vi "Circle_Geometry_Template.vi"(4 "Radius":dbl) -> (0 "Area":dbl, 1 "Circumference":dbl, 2 "Diameter":dbl)   [LabVIEW 2013]
panel:
  # "Circle Geometery\n\nCreate a VI that takes the radius of a circle as an input and\n computes the Diameter, Circumference and Area the circle."
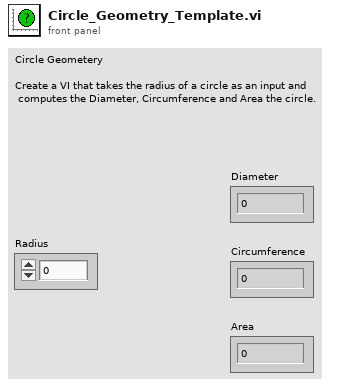
[diagram p1: front panel]
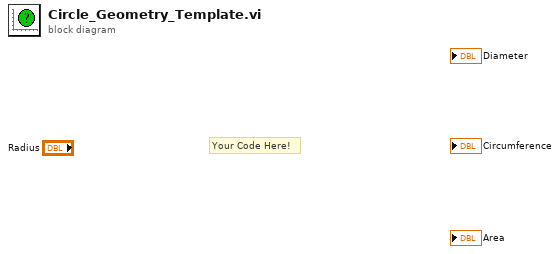
[diagram p0: block diagram]
diagram:
  # "Your Code Here!"
